vi "ConnectionQuality.vi"(11 "Error?":bool) -> (1 "Last Update":timestamp, 3 "Connection Quality":dbl)   [LabVIEW 2017, in "Client.lvlib" / "CommsServer.lvlib"]
uses:
  CommsServer.lvlib
  NI_PtbyPt.lvlib
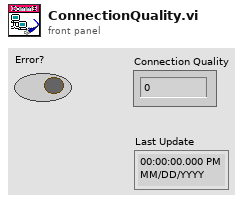
[diagram p1: front panel]
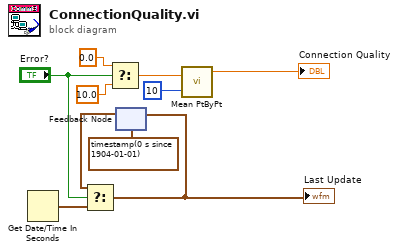
[diagram p0: block diagram]
diagram:
  n1 = Get Date/Time In Seconds() -> (seconds since 1Jan1904=w5:timestamp)
  n2 = Select(t=0.0, s="Error?", f=10.0) -> (s? t:f=w7:dbl)
  n3 = feedback #1(timestamp(0 s since 1904-01-01) ("seconds since 1Jan1904")) -> (w3:timestamp)
  n4 = Select(t=w3, s="Error?", f=w5) -> (s? t:f=w4:timestamp)
  "Last Update" <- w4
  n5 = feedback-in #1(w4) -> ()
  n6 = call "Mean PtByPt.vi"("x"=w7, "sample length"=10) -> ("mean"=→"Connection Quality":dbl)  [unwired: 2 in, 1 out]
